vi "SUB-BLE Rx data save.vi"(4 "Rx Packet Structure":T1={"Message Type (Response)"=128, "Payload length"=25, "Command Class (System)"=4, "Message ID"=5, "Connection handle"=0, "Attribute handle"=11, "Attribute type"=1, "Attribute value (data)"=[18, 16, 0, 0, 255, 1, 84, 254, 142, 65, 148, 2, 57, 254, 79, 254, 141, 128, 14, 213]} {"Attribute type" format="%02x" items=["read", "notify", "indicate", "read_by_type", "read_blob", "indicate_rsp_req"]; "Attribute value (data)" format="%02x"; "Attribute handle" format="%04x"; "Connection handle" format="%02x"; "Message ID" format="%02x"; "Message Type (Response)" format="%02x" items=["Command / Response"=0, "Event"=128]; "Command Class (System)" format="%02x" items=["System", "Persistent Store", "Attribute database", "Connection", "Attribute client", "Security Manager", "Generic Access Profile", "Hardware"]}, 5 "BLE RxD":u8[](array[numeric])) -> (0 "Full packet":u8[](array[numeric]), 1 "Set Packet?":bool, 2 "Mon Packet?":bool)   [LabVIEW 2015]
doc: "Use this template to create an application that executes repeatedly until you click the Stop button. This template polls the state of the Stop button and does not use events. Use the Top-Level Application template (not available in the Base package) to create a single-loop application with event handling."
uses:
  Control-BLED Rx (EVENT-Attribute Client).ctl
  Lib_Bled112 toolkit/type_def/message_type.ctl
  Lib_Bled112 toolkit/type_def/message_class.ctl
  Global 1.vi
panel:
  out "Rx Packet Structure 2":T1={"Message Type (Response)"=128, "Payload length"=0, "Command Class (System)"=1, "Message ID"=0, "Connection handle"=0, "Attribute handle"=0, "Attribute type"=1, "Attribute value (data)"=[]} {"Attribute type" format="%02x" items=["read", "notify", "indicate", "read_by_type", "read_blob", "indicate_rsp_req"]; "Attribute value (data)" format="%02x"; "Attribute handle" format="%04x"; "Connection handle" format="%02x"; "Message ID" format="%02x"; "Message Type (Response)" format="%02x" items=["Command / Response"=0, "Event"=128]; "Command Class (System)" format="%02x" items=["System", "Persistent Store", "Attribute database", "Connection", "Attribute client", "Security Manager", "Generic Access Profile", "Hardware"]}
  # "BLE 수신 데이터 처리: 수신 버퍼에 저장."
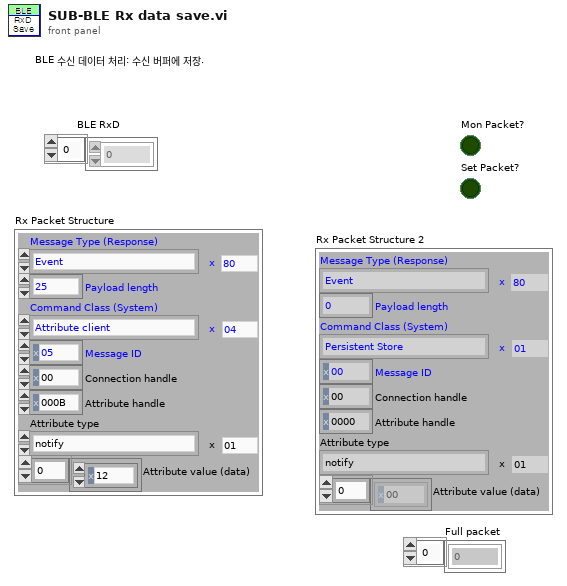
[diagram p1: front panel]
types:
  T1 = typedef "Control-BLED Rx (EVENT-Attribute Client).ctl" = cluster{"Message Type (Response)":T2, "Payload length":u8, "Command Class (System)":T3, "Message ID":u8, "Connection handle":u8, "Attribute handle":u16, "Attribute type":T3, "Attribute value (data)":u8[]}
  T2 = typedef "message_type.ctl" = u8
  T3 = typedef "message_class.ctl" = u8
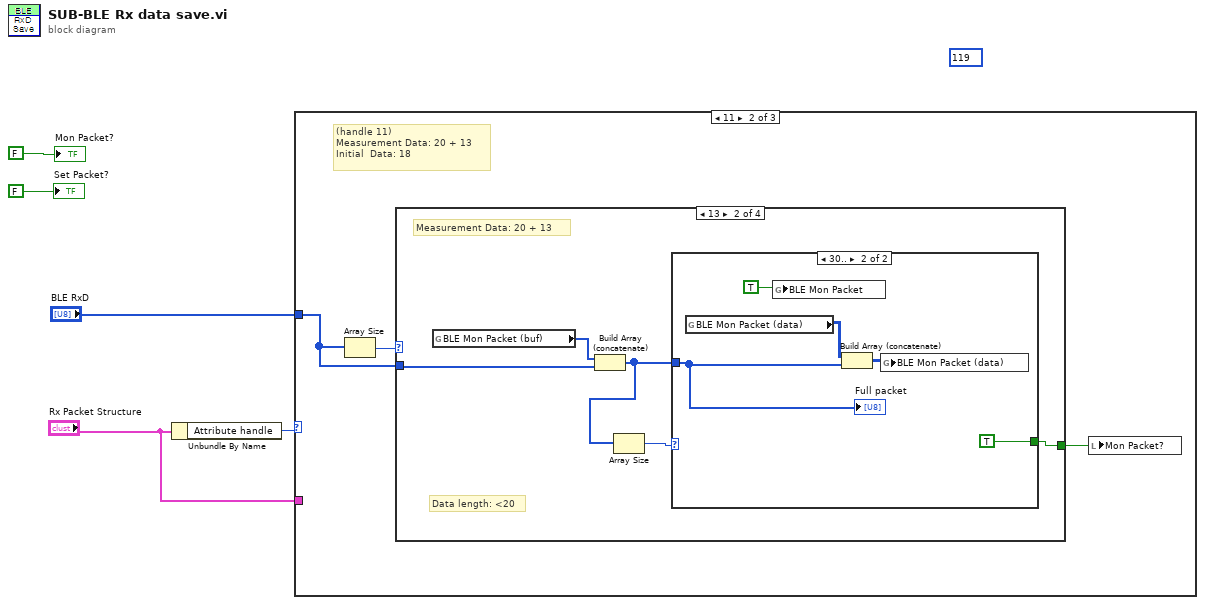
[diagram p0: block diagram]
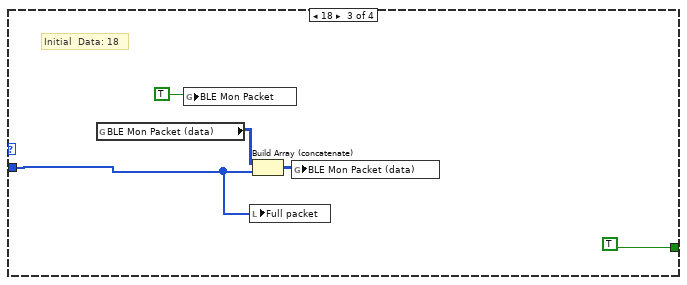
[diagram p5: hidden frame]
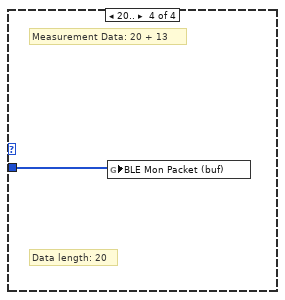
[diagram p6: hidden frame]
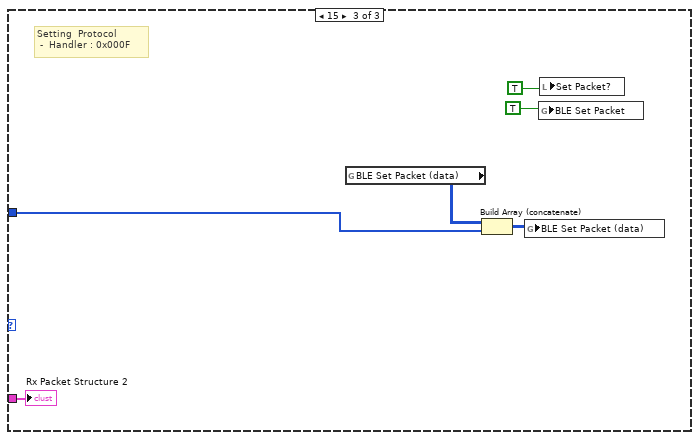
[diagram p7: hidden frame]
diagram:
  (unwired) 119
  n1 = Unbundle By Name("Rx Packet Structure") -> ("Attribute handle"=w4:u16)
  n2 = case shown="11" w4 {
    tunnel: "BLE RxD" -> [_ w7 w26]
    tunnel: "Rx Packet Structure" -> [_ _ w25]
    frame 0, Default {
    }
    frame 11 {
      # "(handle 11)\nMeasurement Data: 20 + 13\nInitial  Data: 18"
      n3 = Array Size(array=w7) -> (size(s)=w8:i32)
      n4 = case shown="13" w8 {
        tunnel: w7 -> [_ w10 w20 w24]
        tunnel: [_ w9 TRUE ("BLE Packet") _] -> w6
        frame 0, Default {
        }
        frame 13 {
          # "Data length: <20"
          # "Measurement Data: 20 + 13"
          n5 = global read "Global 1.vi" "BLE Mon Packet (buf)"() -> (w13:u8[])
          n6 = Build Array (concatenate)(w13, w10) -> (w12:u8[])
          n7 = Array Size(array=w12) -> (size(s)=w11:i32)
          n8 = case shown="30.." w11 {
            tunnel: [_ TRUE ("BLE Packet")] -> w9
            tunnel: w12 -> [_ w14]
            frame 0, Default {
            }
            frame 30.. {
              n9 = global read "Global 1.vi" "BLE Mon Packet (data)"() -> (w17:u8[][])
              n10 = global write "Global 1.vi" "BLE Mon Packet"(TRUE ("BLE Packet")) -> ()
              n11 = Build Array (concatenate)(w17, w14) -> (w16:u8[][])
              n12 = global write "Global 1.vi" "BLE Mon Packet (data)"(w16) -> ()
              "Full packet" <- w14
            }
          }
        }
        frame 18 {
          # "Initial  Data: 18"
          n13 = global read "Global 1.vi" "BLE Mon Packet (data)"() -> (w22:u8[][])
          n14 = global write "Global 1.vi" "BLE Mon Packet"(TRUE ("BLE Packet")) -> ()
          n15 = local write "Full packet"(w20) -> ()
          n16 = Build Array (concatenate)(w22, w20) -> (w21:u8[][])
          n17 = global write "Global 1.vi" "BLE Mon Packet (data)"(w21) -> ()
        }
        frame 20.. {
          # "Data length: 20"
          # "Measurement Data: 20 + 13"
          n18 = global write "Global 1.vi" "BLE Mon Packet (buf)"(w24) -> ()
        }
      }
      n19 = local write "Mon Packet?"(w6) -> ()
    }
    frame 15 {
      # "Setting  Protocol\n - \tHandler : 0x000F"
      n20 = global read "Global 1.vi" "BLE Set Packet (data)"() -> (w28:u8[][])
      n21 = Build Array (concatenate)(w28, w26) -> (w27:u8[][])
      n22 = global write "Global 1.vi" "BLE Set Packet (data)"(w27) -> ()
      n23 = global write "Global 1.vi" "BLE Set Packet"(TRUE ("BLE Packet")) -> ()
      n24 = local write "Set Packet?"(TRUE ("BLE Packet")) -> ()
      "Rx Packet Structure 2" <- w25
    }
  }
  "Mon Packet?" <- FALSE ("Mon Packet?")
  "Set Packet?" <- FALSE ("Set Packet?")
